vi "Unregister Nested.vi"(8 "error in (no error)":errorcluster, 10 "MessageQ":refnum<class "MessageQ.lvclass">, 11 "Module in":refnum<class "Module.lvclass">) -> (0 "error out":errorcluster, 3 "Module out":refnum<class "Module.lvclass">)   [LabVIEW 2020, in "Volatus.lvlib" / "Module.lvclass"]
uses:
  Module.lvclass
  MessageQ/MessageQ.lvclass
  Module.lvclass/Module.ctl
  State.ctl
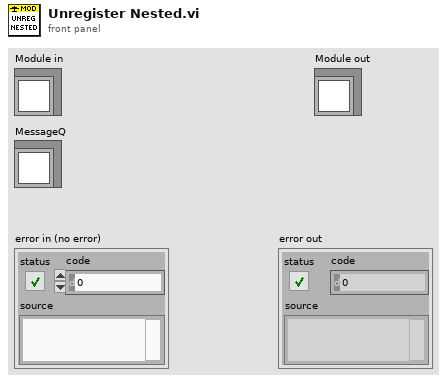
[diagram p1: front panel]
types:
  T1 = typedef "Volatus.lvlib/Module Status.ctl" = cluster{"MessageQ":refnum<class "MessageQ.lvclass">, "State":T2, "Hierarchy":string[]}
  T2 = typedef "Volatus.lvlib/Module.lvclass/State.ctl" = enum16{"Unknown", "Launched", "Starting", "Running", "Stopping", "Stopped", "Error - Starting", "Error - Run", "Error - Stopping"}
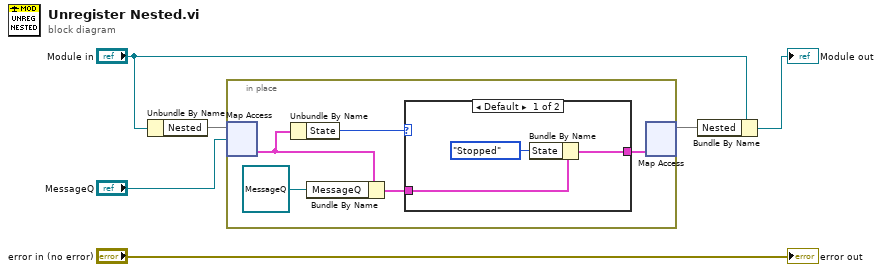
[diagram p0: block diagram]
diagram:
  n1 = Unbundle By Name("Module in") -> ("Nested"=w4:map{refnum<class "MessageQ.lvclass">, T1})
  n2 = in-place {
    n3 = in-place-map #1(w4, "MessageQ") -> (w10:T1)  [unwired: 1 in, 1 out]
    n4 = Unbundle By Name(w10) -> ("State"=w8:T2)
    n5 = Bundle By Name(cluster=w10, "MessageQ"=refnum<class "MessageQ.lvclass"> refnum) -> (w9:T1)
    n6 = case shown="Default" w8 {
      tunnel: w9 -> [w14 w15]
      tunnel: [w12 w15] -> w7
      frame Default {
        n7 = Bundle By Name(cluster=w14, "State"=State."Stopped") -> (w12:T1)
      }
      frame "Error - Starting".."Error - Stopping" {
      }
    }
    n8 = in-place-map #1(w7) -> (w2:map{refnum<class "MessageQ.lvclass">, T1})  [unwired: 1 in, 2 out]
  }
  n9 = Bundle By Name(cluster="Module in", "Nested"=w2) -> (→"Module out":refnum<class "Module.lvclass">)
  "error out" <- "error in (no error)"
